vi "OCV 4309 Finite.vi"(8 "error in":errorcluster, 10 "Rate (Hz)":dbl=1000.0 format="%#_13g") -> (0 "error out":errorcluster, 1 "Elapsed Time (ms)":u32=1599, 2 "Results":T1)   [LabVIEW 2019]
doc: "This example demonstrates how to enable the Chop feature in a continuously acquire buffered voltage measurement using a DAQmx device.\n\nFor instructions on how to connect your signals to the DAQ device, refer to your device documentation."
uses:
  labview-grpc-query-server/VIs/MeasurementServer_OCVRawData.ctl
  labview-grpc-query-server/VIs/MeasurementServer_ErrorOutData.ctl
  <vilib>/DAQmx/read.llb/DAQmx Read (Analog 1D DBL NChan 1Samp).vi
  <vilib>/DAQmx/create/channels.llb/DAQmx Create Channel (AI-Voltage-Basic).vi
  <vilib>/DAQmx/configure/timing.llb/DAQmx Timing (Sample Clock).vi
  <vilib>/DAQmx/miscellaneous.llb/DAQmx Fill In Error Info.vi
  <resource>/objmgr/daqmx.rc
  labview-grpc-query-server/VIs/labview-grpc-measurement-server.lvlib
panel:
  out "Voltage":dbl[](array[numeric]) format="%#_8g"
  in  "Chop":bool=TRUE
  in  "Max Voltage":dbl=10.0
  in  "Min Voltage":dbl=-10.0
  in  "Physical Channel":tag="4309/ai0:4"
  # "DAQmx Settings"
  # "On (T)"
  # "Off (F)"
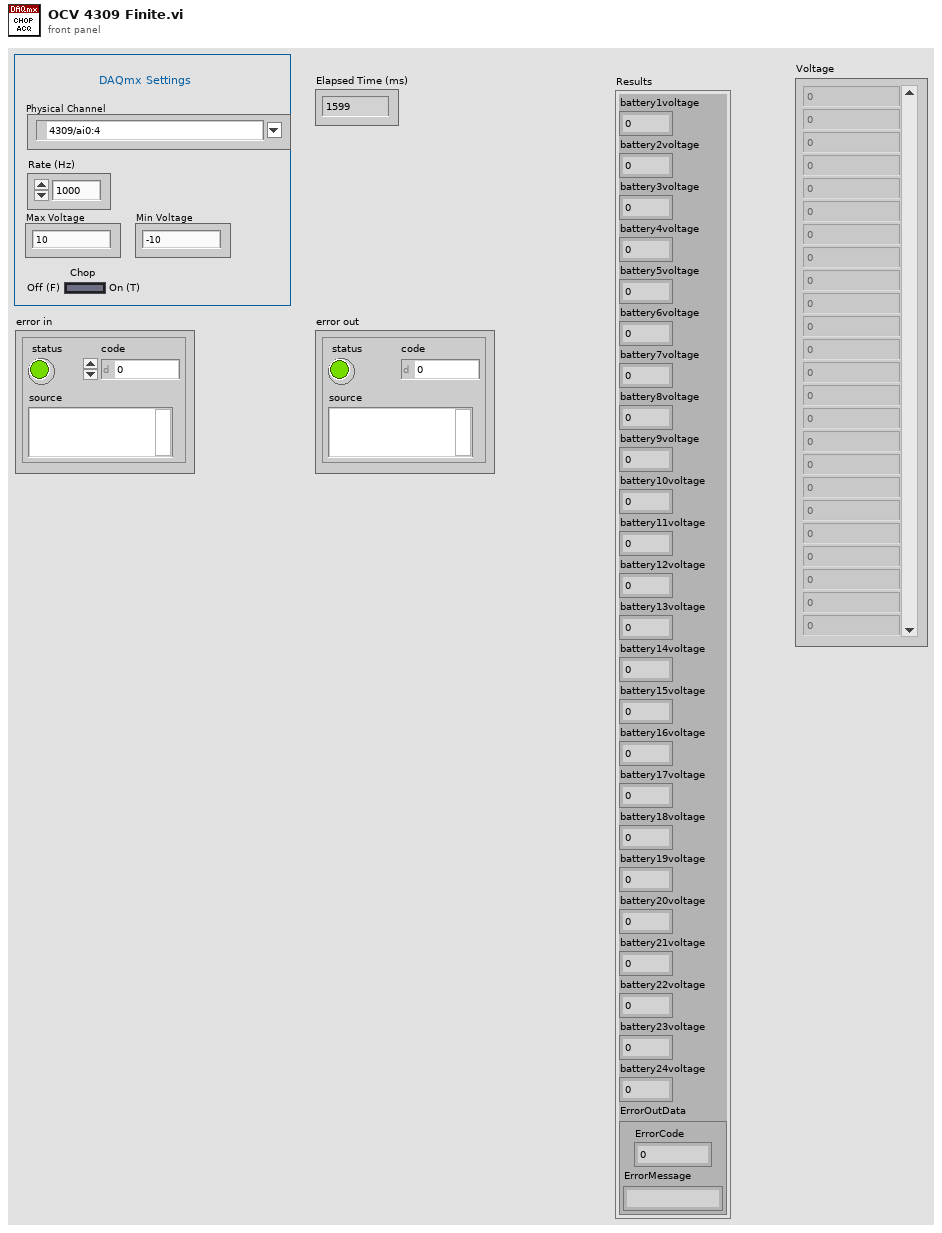
[diagram p1: front panel]
types:
  T1 = typedef "labview-grpc-measurement-server.lvlib/MeasurementServer_OCVRawData.ctl" = cluster{"battery1voltage":sgl, "battery2voltage":sgl, "battery3voltage":sgl, "battery4voltage":sgl, "battery5voltage":sgl, "battery6voltage":sgl, "battery7voltage":sgl, "battery8voltage":sgl, "battery9voltage":sgl, "battery10voltage":sgl, "battery11voltage":sgl, "battery12voltage":sgl, "battery13voltage":sgl, "battery14voltage":sgl, "battery15voltage":sgl, "battery16voltage":sgl, "battery17voltage":sgl, "battery18voltage":sgl, "battery19voltage":sgl, "battery20voltage":sgl, "battery21voltage":sgl, "battery22voltage":sgl, "battery23voltage":sgl, "battery24voltage":sgl, "ErrorOutData":T2}
  T2 = typedef "labview-grpc-measurement-server.lvlib/MeasurementServer_ErrorOutData.ctl" = cluster{"ErrorCode":i32, "ErrorMessage":string}
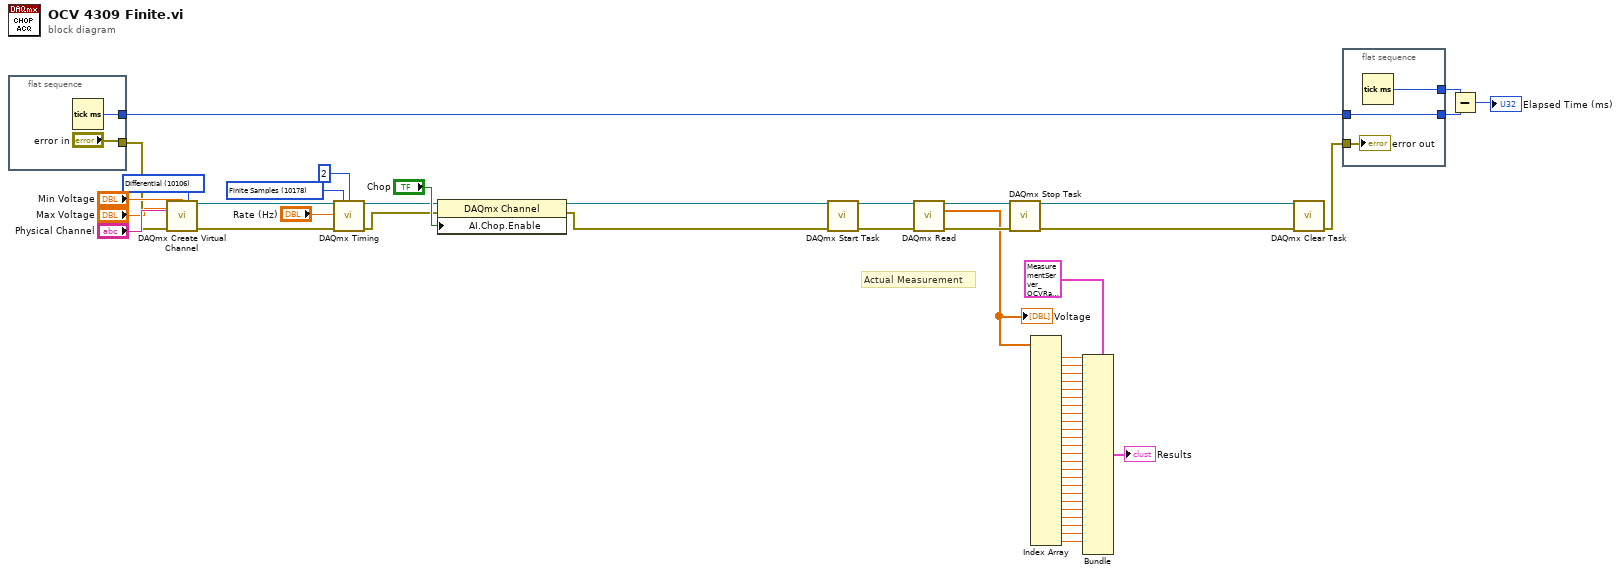
[diagram p0: block diagram]
diagram:
  w52 = 10106 items=["default"=-1, "RSE"=10083, "NRSE"=10078, "Differential"=10106, "Pseudodifferential"=12529] ("Terminal Configuration")
  w39 = 10178 items=["Finite Samples"=10178, "Continuous Samples"=10123, "Hardware Timed Single Point"=12522] ("sample mode")
  # "Actual Measurement"
  n1 = flat-sequence {
    tunnel: [w55] -> w34
    tunnel: ["error in"] -> w29
    frame #0 {
      n2 = Tick Count (ms)() -> (millisecond timer value=w55:u32)
    }
  }
  n3 = call-poly <vilib>:"DAQmx Create Virtual Channel.vi"("maximum value"="Max Voltage", "minimum value"="Min Voltage", "input terminal configuration"=w52, "physical channels"="Physical Channel", "error in"=w29) -> ("task out"=w43:refnum<k21>, "error out"=w46:errorcluster)  [unwired: 9 in]
  n4 = call-poly <vilib>:"DAQmx Timing.vi"("task/channels in"=w43, "sample mode"=w39, "samples per channel"=2, "rate"="Rate (Hz)", "error in"=w46) -> ("task out"=w44:refnum<k21>, "error out"=w45:errorcluster)  [unwired: 9 in]
  n5 = property class="DAQmx Channel"(reference=w44, error in=w45, "AI.Chop.Enable"="Chop") -> (reference out=w42:refnum<k21>, error out=w41:errorcluster)
  n6 = call <vilib>:"DAQmx Start Task.vi"("task/channels in"=w42, "error in"=w41) -> ("task out"=w32:refnum<k21>, "error out"=w31:errorcluster)  [unwired: 12 in]
  n7 = call-poly <vilib>:"DAQmx Read.vi"("task/channels in"=w32, "error in"=w31) -> ("task out"=w36:refnum<k21>, "data"=w20:dbl[], "error out"=w37:errorcluster)  [unwired: 11 in]
  "Voltage" <- w20
  n8 = call <vilib>:"DAQmx Stop Task.vi"("task/channels in"=w36, "error in"=w37) -> ("task out"=w48:refnum<k21>, "error out"=w49:errorcluster)  [unwired: 12 in]
  n9 = Index Array(array=w20) -> (element #1=w25:dbl, element #2=w24:dbl, element #3=w23:dbl, element #4=w22:dbl, element #5=w21:dbl, element #6=w19:dbl, element #7=w18:dbl, element #8=w17:dbl, element #9=w16:dbl, element #10=w15:dbl, element #11=w14:dbl, element #12=w13:dbl, element #13=w12:dbl, element #14=w11:dbl, element #15=w10:dbl, element #16=w9:dbl, element #17=w8:dbl, element #18=w7:dbl, element #19=w6:dbl, element #20=w5:dbl, element #21=w4:dbl, element #22=w3:dbl, element #23=w2:dbl, element #24=w1:dbl)  [unwired: 24 in]
  n10 = Bundle(cluster=T1 {"battery1voltage"=0.0, "battery2voltage"=0.0, "battery3voltage"=0.0, "battery4voltage"=0.0, "battery5voltage"=0.0, "battery6voltage"=0.0, "battery7voltage"=0.0, "battery8voltage"=0.0, "battery9voltage"=0.0, "battery10voltage"=0.0, "battery11voltage"=0.0, "battery12voltage"=0.0, "battery13voltage"=0.0, "battery14voltage"=0.0, "battery15voltage"=0.0, "battery16voltage"=0.0, "battery17voltage"=0.0, "battery18voltage"=0.0, "battery19voltage"=0.0, "battery20voltage"=0.0, "battery21voltage"=0.0, "battery22voltage"=0.0, "battery23voltage"=0.0, "battery24voltage"=0.0, "ErrorOutData"={"ErrorCode"=0, "ErrorMessage"=""}} ("OCVRawData in"), "battery1voltage"=w25, "battery2voltage"=w24, "battery3voltage"=w23, "battery4voltage"=w22, "battery5voltage"=w21, "battery6voltage"=w19, "battery7voltage"=w18, "battery8voltage"=w17, "battery9voltage"=w16, "battery10voltage"=w15, "battery11voltage"=w14, "battery12voltage"=w13, "battery13voltage"=w12, "battery14voltage"=w11, "battery15voltage"=w10, "battery16voltage"=w9, "battery17voltage"=w8, "battery18voltage"=w7, "battery19voltage"=w6, "battery20voltage"=w5, "battery21voltage"=w4, "battery22voltage"=w3, "battery23voltage"=w2, "battery24voltage"=w1) -> (→"Results":T1)  [unwired: 1 in]
  n11 = call <vilib>:"DAQmx Clear Task.vi"("task in"=w48, "error in"=w49) -> ("error out"=w28:errorcluster)  [unwired: 13 in]
  n12 = flat-sequence {
    tunnel: w28 -> [w57]
    tunnel: [w58] -> w35
    tunnel: w34 -> [w56]
    tunnel: [w56] -> w33
    frame #0 {
      n13 = Tick Count (ms)() -> (millisecond timer value=w58:u32)
      "error out" <- w57
    }
  }
  n14 = Subtract(x=w35, y=w33) -> (x-y=→"Elapsed Time (ms)":u32)
